vi "Read TDMS Wavenames into Ring.vi"(8 "error in (no error)":errorcluster, 10 "Ring Refs []":refnum<vi>[](array[refnum]), 11 "File or Folder Path":path=path "C:/") -> (0 "error out":errorcluster)   [LabVIEW 2016, in "LV-Data.TDMS.lvclass"]
uses:
  LV-Data.TDMS.lvclass
  LV-Data/LV-Data.lvclass
panel:
  out "Names []":string[](array[string])
  out "Channels":cluster{"X":u16, "Y":u16, "N":u16} {"N" items=["time", "temp", "B", "AI1", "AI2", "AI3", "AI4", "AI5", "AI6", "AO1", "AO2", "AO3", "AO4"]; "Y" items=["time", "temp", "B", "AI1", "AI2", "AI3", "AI4", "AI5", "AI6", "AO1", "AO2", "AO3", "AO4"]; "X" items=["time", "temp", "B", "AI1", "AI2", "AI3", "AI4", "AI5", "AI6", "AO1", "AO2", "AO3", "AO4"]}
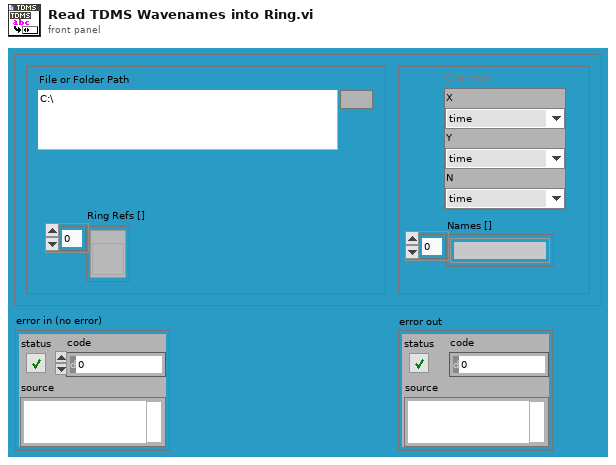
[diagram p1: front panel]
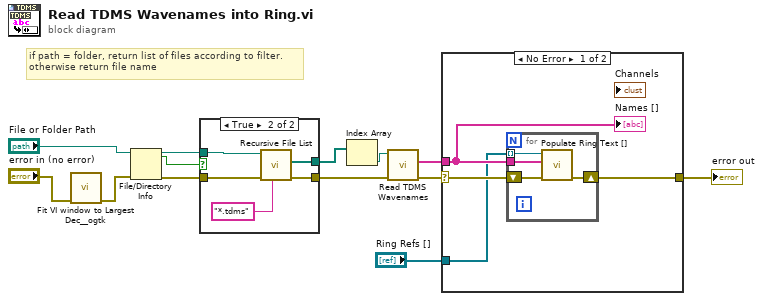
[diagram p0: block diagram]
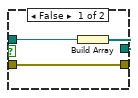
[diagram p3: hidden frame]
diagram:
  # "if path = folder, return list of files according to filter.\notherwise return file name"
  n1 = call <userlib>:"Fit VI window to Largest Dec__ogtk.vi"("error in (no error)"="error in (no error)") -> ("error out"=w7:errorcluster)  [unwired: 5 in, 1 out]
  n2 = File/Directory Info(path="File or Folder Path", error in=w7) -> (path out=w9:path, directory=w11:bool, error out=w10:errorcluster)  [unwired: 4 out]
  n3 = case shown="True" w11 {
    tunnel: [w16 w20] -> w3
    tunnel: w9 -> [w15 w21]
    tunnel: w10 -> [w14 w19]
    tunnel: [w14 w18] -> w12
    frame False {
      n4 = Build Array(w15) -> (w16:path[])
    }
    frame True {
      n5 = call <vilib>:"Recursive File List.vi"("pattern"="*.tdms", "error in (no error)"=w19, "Folder Path"=w21) -> ("error out"=w18:errorcluster, "All Files in Dir"=w20:path[])  [unwired: 4 in, 3 out]
    }
  }
  n6 = Index Array(array=w3) -> (element=w1:path)  [unwired: 1 in]
  n7 = call "Read TDMS Wavenames.vi"("error in (no error)"=w12, "path"=w1) -> ("error out"=w5:errorcluster, "Wavenames"=w6:string[])  [unwired: 7 in, 1 out]
  n8 = case shown="No Error" w5 {
    selector: w5 -> [w25 w30]
    tunnel: w6 -> [w24 _]
    tunnel: [w23 w30] -> w4
    tunnel: "Ring Refs []" -> [w22 _]
    frame No Error {
      n9 = for {
        tunnel: w24 -> [w28]
        shift-right: [w27] -> w23
        shift-left: w25 -> [w29]
        tunnel: w22 -> [w26] mode=indexing
        n10 = call "Populate Ring Text [].vi"("error in (no error)"=w29, "Strings []"=w28, "Ring in"=w26) -> ("error out"=w27:errorcluster)  [unwired: 8 in]
      }
      "Names []" <- w24
    }
    frame Error {
    }
  }
  "error out" <- w4
